vi "BRig_dataExp_LaserSwitch_Prob_l1.vi"() -> (2 "output_LaserSwitch_Probability_L1":i32)   [LabVIEW 2014]
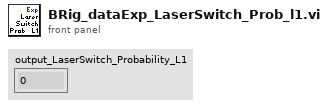
[diagram p1: front panel]
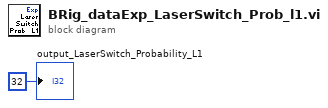
[diagram p0: block diagram]
diagram:
  "output_LaserSwitch_Probability_L1" <- 32 ("output_iBlock")
